vi "LAB1.vi"() -> ()   [LabVIEW 2018]
doc: "zamiana temperatury w skali f w skalê K lub C"
panel:
  out "Alarm":bool
  in  "Tkryt":dbl
  out "Waveform Chart":dbl(graph)
  in  "stop":bool
  in  "TK/TC":bool
  out "TK/TC":dbl
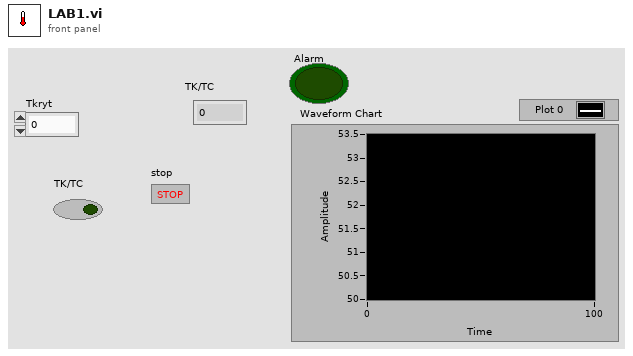
[diagram p1: front panel]
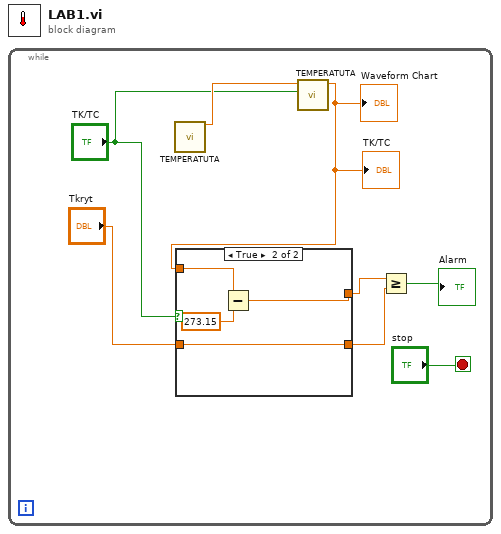
[diagram p0: block diagram]
diagram:
  n1 = while {
    stop <- "stop" stop-if-true
    n2 = call "TEMPERATUTA.vi"() -> ("T (F)"=w6:dbl)  [unwired: 15 in]
    n3 = call "TEMPERATUTA.vi"("TK/TC"="TK/TC", "Tf"=w6) -> ("TC"=w1:dbl)  [unwired: 9 in]
    "TK/TC" <- w1
    "Waveform Chart" <- w1
    n4 = case shown="True" "TK/TC" {
      tunnel: "Tkryt" -> [w10 w11]
      tunnel: [w9 w12] -> w3
      tunnel: [w10 w11] -> w5
      tunnel: w1 -> [w9 w14]
      frame False {
      }
      frame True {
        n5 = Subtract(x=w14, y=273.15 ("x-y")) -> (x-y=w12:dbl)
      }
    }
    n6 = Greater Or Equal?(x=w3, y=w5) -> (x >= y?=→"Alarm":bool)
  }
